vi "PolInterpret.vi"(2 "Format":enum16{"ASCII", "Binary"}(ring)=enum."Binary", 3 "Time Bytes Before Output":i32, 4 "#Bytes":i32[](array[numeric])=[3, 4, 4, 4, 4, 4, 4, 3, 4, 4, 4, 4, 4, 4, 2], 5 "Polhemus Output":string) -> (0 "Interpreted Values":sgl[](array[numeric]), 1 "Time":i32)   [LabVIEW 2012]
doc: "Takes direct output from the Polhemus (+7 bytes preceding for timing), and uses information about the number of bytes per piece in the output to construct a set of interpreted values."
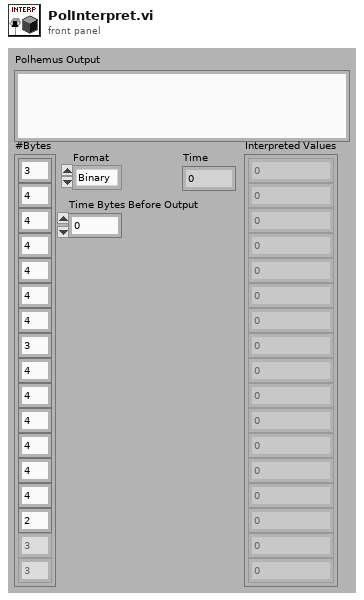
[diagram p1: front panel]
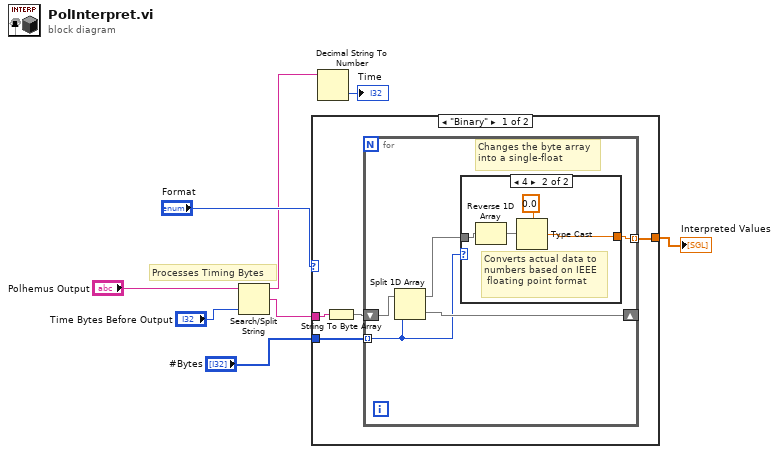
[diagram p0: block diagram]
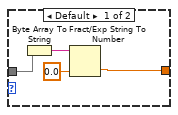
[diagram p2: hidden frame]
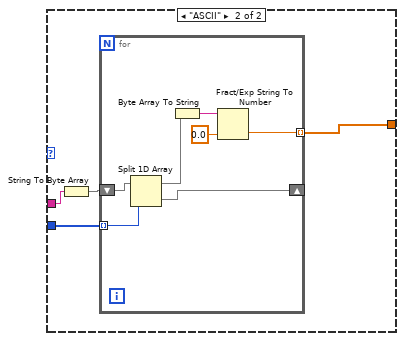
[diagram p3: hidden frame]
diagram:
  # "Processes Timing Bytes"
  n1 = Search/Split String(string="Polhemus Output", offset (0)="Time Bytes Before Output") -> (substring before match=w5:string, match + rest of string=w3:string)  [unwired: 1 in, 1 out]
  n2 = case shown="\"Binary\"" "Format" {
    tunnel: w3 -> [w11 w28]
    tunnel: "#Bytes" -> [w12 w29]
    tunnel: [w9 w26] -> w7
    frame "Binary" {
      n3 = String To Byte Array(string=w11) -> (unsigned byte array=w10:u8[])
      n4 = for {
        tunnel: w12 -> [w15] mode=indexing
        shift-right: [w16] -> _
        shift-left: w10 -> [w17]
        tunnel: [w13] -> w9 mode=indexing
        # "Changes the byte array\ninto a single-float"
        n5 = Split 1D Array(array=w17, index=w15) -> (first subarray=w14:u8[], second subarray=w16:u8[])
        n6 = case shown="4" w15 {
          tunnel: w14 -> [w19 w23]
          tunnel: [w18 w24] -> w13
          frame Default {
            n7 = Byte Array To String(unsigned byte array=w19) -> (string=w21:string)
            n8 = Fract/Exp String To Number(string=w21, default (0 dbl)=sgl 0.0 ("default (0 I32)")) -> (number=w18:sgl)  [unwired: 2 in, 1 out]
          }
          frame 4 {
            # "Converts actual data to\nnumbers based on IEEE\n floating point format"
            n9 = Reverse 1D Array(array=w23) -> (reversed array=w22:u8[])
            n10 = Type Cast(type=sgl 0.0, x=w22) -> (*(type *) &x=w24:sgl)
          }
        }
      }
    }
    frame "ASCII" {
      n11 = String To Byte Array(string=w28) -> (unsigned byte array=w27:u8[])
      n12 = for {
        tunnel: w29 -> [w34] mode=indexing
        shift-right: [w35] -> _
        shift-left: w27 -> [w36]
        tunnel: [w30] -> w26 mode=indexing
        n13 = Split 1D Array(array=w36, index=w34) -> (first subarray=w33:u8[], second subarray=w35:u8[])
        n14 = Byte Array To String(unsigned byte array=w33) -> (string=w32:string)
        n15 = Fract/Exp String To Number(string=w32, default (0 dbl)=sgl 0.0 ("default (0 I32)")) -> (number=w30:sgl)  [unwired: 2 in, 1 out]
      }
    }
  }
  "Interpreted Values" <- w7
  n16 = Decimal String To Number(string=w5) -> (number=→"Time":i32)  [unwired: 2 in, 1 out]
